vi "Constants.vi"() -> ()   [LabVIEW 2015, in "Control Addon Shared.lvlib"]
doc: "Use this Global VI to access the GUIDs assigned to the page resources of the Custom Device."
uses:
  Control Addon Shared.lvlib
panel:
  in  "Tab Control":enum32{"GUIDS", "Constants", "Properties"}(tab)=enum."Constants"
  in  "GUID.IndustrialManualState":string="08f692c4-1545-427d-bddb-8fc3035cef48"
  in  "GUID.IndustrialParameters":string="96a5c8c8-4405-4e2d-832c-ba7077f33cb8"
  in  "GUID.IndustrialController":string="c3f6d8cf-9ad7-4a46-8584-d15a442091f1"
  in  "GUID.ControlDisable":string="dbd079b4-f3f8-48b6-80e4-b86baf99072c"
  in  "GUID.Setpoint":string="45cf5b34-ee61-4dc1-a452-b5ea301868c0"
  in  "GUID.Output":string="d712e0d2-113f-4ca0-b313-0b238ae04ab3"
  in  "GUID.PIDManualOutput":string="33e1e162-1383-425c-bdb7-427d30bbaf11"
  in  "GUID.Channels":string="0e9f6a7a-1f60-42ed-aebc-7ade1398e17a"
  in  "GUID.ManualControl":string="3c58b7de-1473-49f6-b484-be00c9625176"
  in  "GUID.PIDParameters":string="1cc989ca-4b2f-491b-ac05-844f3fc006dc"
  in  "GUID.PIDController":string="a4932adc-e764-4f49-9467-a4fe8850f52e"
  in  "GUID.Control":string="8dfd0406-1a5d-45dd-a1d7-1d4d9090bfa4"
  in  "Controller.RateLimiter":string="RateLimiter"
  in  "Name.IndustrialManualState":string="Manual State"
  in  "Name.IndustriaParameters":string="Industrial Parameters"
  in  "Name.IndustrialController":string="Industrial Controller"
  in  "IndustrialParameters.MinimumSwitchingDuration":string="MinimumSwitchingDuration"
  in  "IndustrialParameters.EnableSwitchingFilter":string="EnableSwitchingFilter"
  in  "IndustrialParameters.SetpointHysteresis":string="SetpointHysteresis"
  in  "IndustrialParameters.EnableSetpointHysteresis":string="EnableSetpointHysteresis"
  in  "Main.CompiledSettings":string="CompiledSettings"
  in  "Name.PIDManualOutput":string="Manual Output"
  in  "Name.ManualControl":string="Manual Control"
  in  "PIDParameters.PIDArray":string="PIDArray"
  in  "PIDParameters.EnableLiveUpdates":string="EnableLiveUpdates"
  in  "PIDParameters.EnableGainScheduling":string="EnableGainScheduling"
  in  "PIDParameters.GainScheduleNode":string="GainScheduleNode"
  in  "Name.Channels":string="Channels"
  in  "Name.Output":string="Output"
  in  "Name.Setpoint":string="Setpoint"
  in  "Name.PIDParameters":string="PID Parameters"
  in  "Name.PIDController":string="PID Controller"
  in  "Name.SimplePID":string="Simple PID"
  in  "Controller.ExternalSetpoint":string="ExternalSetpoint"
  in  "Controller.SetpointMax":string="SetpointMax"
  in  "Controller.SetpointMin":string="SetpointMin"
  in  "Controller.OutputMin":string="OutputMin"
  in  "Controller.OutputMax":string="OutputMax"
  in  "Controller.OutputNode":string="OutputNode"
  in  "Controller.SetpointNode":string="SetpointNode"
  in  "Controller.FeedbackNode":string="FeedbackNode"
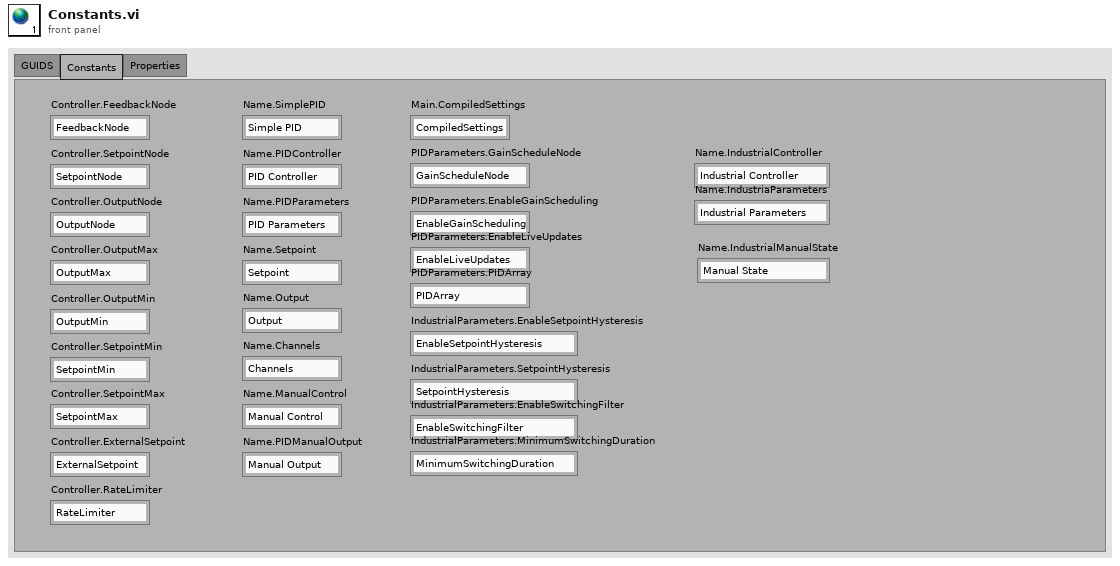
[diagram p1: front panel]
diagram:
